vi "X_Read From XML File(string).vi"(5 "pattern (*.xml)":string="*.xml", 7 "Prompt":string="Select Path to XML File", 8 "error in (no error)":errorcluster, 11 "XML File Path":path) -> (0 "error out":errorcluster, 2 "XML Elements":string, 3 "XML File Path(duplicate)":path)   [LabVIEW 2021, in "Files.lvlib"]
doc: "Reads and parses tags from a LabVIEW XML file. When you place this VI on the block diagram, the polymorphic VI selector is visible. Use this selector to choose which polymorphic instance to use. All XML data must follow the standard LabVIEW XML schema."
uses:
  Files.lvlib
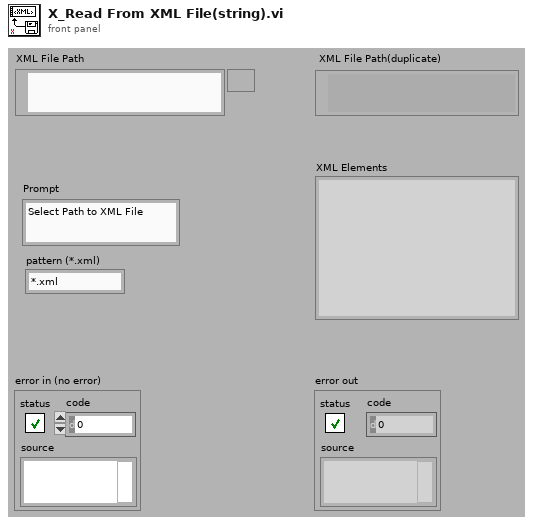
[diagram p1: front panel]
types:
  T1 = enum16{"open", "open or create", "create or replace", "create", "open (read only)"}
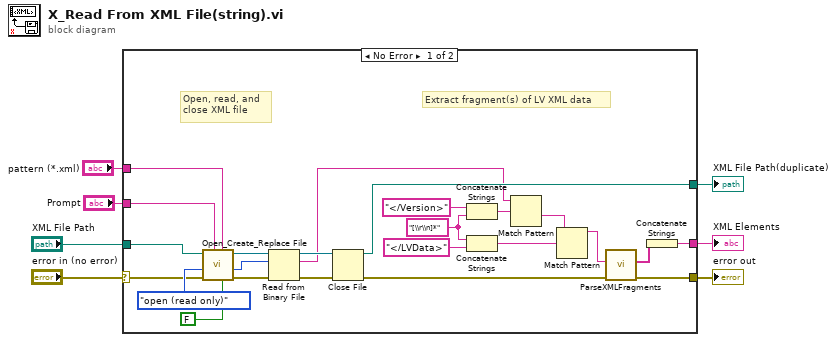
[diagram p0: block diagram]
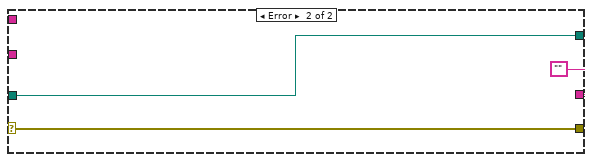
[diagram p2: hidden frame]
diagram:
  n1 = case shown="No Error" "error in (no error)" {
    selector: "error in (no error)" -> [w27 w34]
    tunnel: [w22 w34] -> w6
    tunnel: [w20 w33] -> w5
    tunnel: "XML File Path" -> [w29 w33]
    tunnel: [w18 ""] -> w3
    tunnel: "Prompt" -> [w9 _]
    tunnel: "pattern (*.xml)" -> [w8 _]
    frame No Error {
      w12 = "[\\r\\n]*"
      # "Extract fragment(s) of LV XML data"
      # "Open, read, and \nclose XML file"
      n2 = call <vilib>:"Open_Create_Replace File.vi"("advisory dialog? (display:T)"=FALSE, "pattern"=w8, "prompt"=w9, "error in (no error)"=w27, "function (open:0)"=T1."open (read only)", "file path"=w29) -> ("error out"=w15:errorcluster, "file size (bytes)"=w16:i32, "refnum"=w17:refnum<file>)  [unwired: 2 in, 1 out]
      n3 = Read from Binary File(8:w15, 10:w16, 11:w17) -> (0:w13:errorcluster, 2:w11:string, 3:w14:refnum<file>)  [unwired: 3 in, 1 out]
      n4 = Close File(refnum=w14, error in=w13) -> (path=w20:path, error out=w21:errorcluster)
      n5 = Concatenate Strings("</Version>", w12) -> (w24:string)
      n6 = Concatenate Strings(w12, "</LVData>" ("Substring")) -> (w25:string)
      n7 = Match Pattern(string=w11, regular expression=w24) -> (after substring=w26:string)  [unwired: 1 in, 3 out]
      n8 = Match Pattern(string=w26, regular expression=w25) -> (before substring=w23:string)  [unwired: 1 in, 3 out]
      n9 = call <vilib>:"ParseXMLFragments.vi"("error in (no error)"=w21, "XML in"=w23) -> ("error out"=w22:errorcluster, "XML Elements"=w19:string[])  [unwired: 8 in]
      n10 = Concatenate Strings(w19) -> (w18:string)
    }
    frame Error {
    }
  }
  "error out" <- w6
  "XML File Path(duplicate)" <- w5
  "XML Elements" <- w3
